vi "ErrorBooleanRef.vi"(8 "error in (no error)":errorcluster, 10 "Error Indicator Boolean Ref":refnum<vi>, 11 "object in":refnum<class "EventLogger_Actor.lvclass">) -> (0 "error out":errorcluster, 3 "object out":refnum<class "EventLogger_Actor.lvclass">)   [LabVIEW 2014, in "EventLogger_Actor.lvlib" / "EventLogger_Actor.lvclass"]
uses:
  EventLogger_Actor.lvclass
  EventLogger_Actor.lvclass/EventLogger_Actor.ctl
panel:
  # "BSD 2-Clause License\n\nCopyright (c) 2018, Ajay www.digiajay.com\nAll rights reserved.\n\nRedistribution and use in source and binary forms, with or without\nmodification, are permitted provided that the following conditions are met:\n\n* Redistributions of source code must retain the above copyright notice, this\n  list of conditions and the following disclaimer.\n\n* Redistributions in binary form must reproduce the above copyright notice,\n  this list of conditions and the following disclaimer in the documentation\n  and/or other materials provided with the distribution.\n\nTHIS SOFTWARE IS PROVIDED BY THE COPYRIGHT HOLDERS AND CONTRIBUTORS \"AS IS\"\nAND ANY EXPRESS OR IMPLIED WARRANTIES, INCLUDING, BUT NOT LIMITED TO, THE\nIMPLIED WARRANTIES OF MERCHANTABILITY AND FITNESS FOR A PARTICULAR PURPOSE ARE\nDISCLAIMED. IN NO EVENT SHALL THE COPYRIGHT HOLDER OR CONTRIBUTORS BE LIABLE\nFOR ANY DIRECT, INDIRECT, INCIDENTAL, SPECIAL, EXEMPLARY, OR CONSEQUENTIAL\nDAMAGES (INCLUDING, BUT NOT LIMITED TO, PROCUREMENT OF SUBSTITUTE GOODS OR\nSERVICES; LOSS OF USE, DATA, OR PROFITS; OR BUSINESS INTERRUPTION) HOWEVER\nCAUSED AND ON ANY THEORY OF LIABILITY, WHETHER IN CONTRACT, STRICT LIABILITY,\nOR TORT (INCLUDING NEGLIGENCE OR OTHERWISE) ARISING IN ANY WAY OUT OF THE USE\nOF THIS SOFTWARE, EVEN IF ADVISED OF THE POSSIBILITY OF SUCH DAMAGE."
  # "Connector Pane"
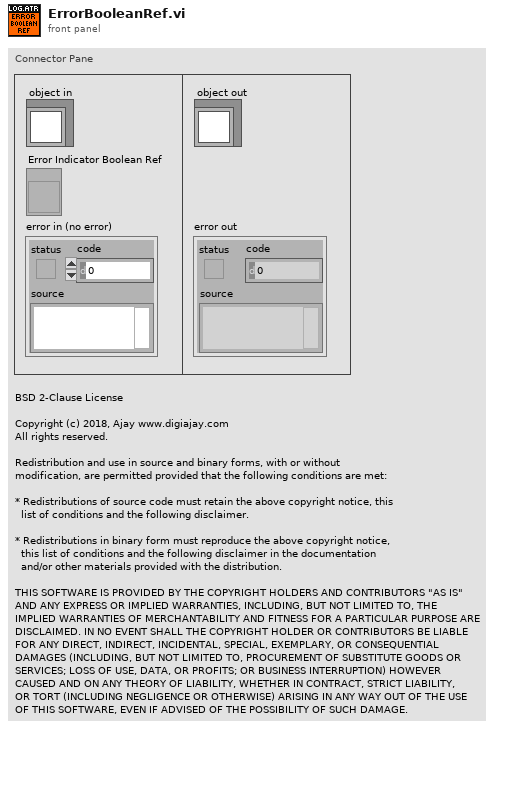
[diagram p1: front panel]
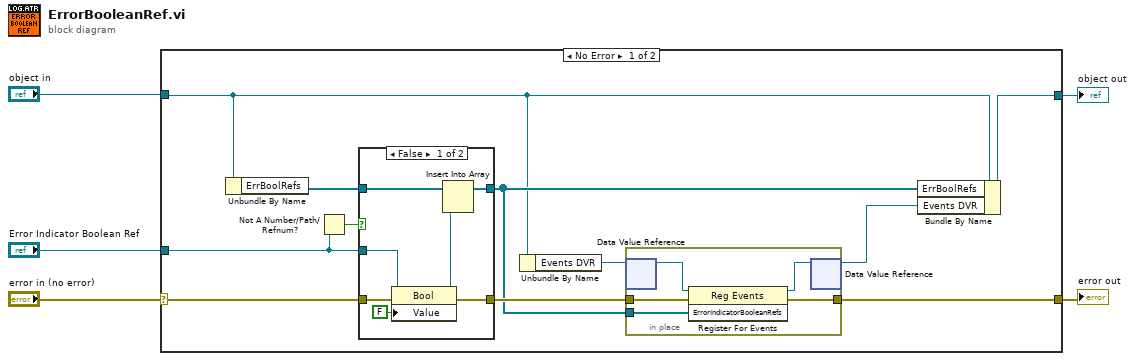
[diagram p0: block diagram]
diagram:
  n1 = case shown="No Error" "error in (no error)" {
    selector: "error in (no error)" -> [w16 w32]
    tunnel: [w10 w32] -> w4
    tunnel: [w15 w31] -> w2
    tunnel: "object in" -> [w7 w31]
    tunnel: "Error Indicator Boolean Ref" -> [w12 _]
    frame No Error {
      n2 = Unbundle By Name(w7) -> ("ErrBoolRefs"=w14:refnum<vi>[])
      n3 = Not A Number/Path/Refnum?(number/path/refnum=w12) -> (NaN/Path/Refnum?=w11:bool)
      n4 = case shown="False" w11 {
        tunnel: w16 -> [w28 w29]
        tunnel: [w27 w30] -> w9
        tunnel: w14 -> [w26 w30]
        tunnel: [w25 w29] -> w13
        tunnel: w12 -> [w22 _]
        frame False {
          n5 = property class="Bool"(reference=w22, error in=w28, "Value"=FALSE) -> (reference out=w24:refnum<vi>, error out=w25:errorcluster)
          n6 = Insert Into Array(array=w26, new element=w24) -> (w27:refnum<vi>[])  [unwired: 1 in]
        }
        frame True {
        }
      }
      n7 = Unbundle By Name(w7) -> ("Events DVR"=w6:refnum<data-value>)
      n8 = in-place {
        in-place-border: w13 -> [w21]
        in-place-border: [w20] -> w10
        in-place-border: w9 -> [w19]
        n9 = in-place-dvr #1(w6) -> (w17:refnum<event-registration>)  [unwired: 1 out]
        n10 = register-events(reference=w17, error in=w21, w19) -> (reference out=w18:refnum<event-registration>, error out=w20:errorcluster)
        n11 = in-place-dvr #1(w18) -> (w8:refnum<data-value>)  [unwired: 1 out]
      }
      n12 = Bundle By Name(cluster=w7, "ErrBoolRefs"=w9, "Events DVR"=w8) -> (w15:refnum<class "EventLogger_Actor.lvclass">)
    }
    frame Error {
    }
  }
  "error out" <- w4
  "object out" <- w2
